vi "Update Settings button colors.vi"(7 "Host":T1, 8 "error in (no error)":errorcluster, 9 "Force Default Colors (F)":bool, 10 "Bool Refnum":refnum<vi>, 11 "Settings in":T4) -> (0 "error out":errorcluster, 3 "Settings out":T4)   [LabVIEW 2021]
doc: "Change the colors of the boolean button according to Settings in and Host in. Consider whether the data log file will be overwritten: default colors when safe, red tint when overwriting. Otherwise, consider whether there are no IO resources: default colors when present, yellow tint when missing."
uses:
  Settings/Settings.lvlib
  Acquisition/IO Device.ctl
  Acquisition/Acquisition.lvlib
  Acquisition/Channel Settings.ctl
  Interval Timer/Interval Length.ctl
  Interval Timer/Interval Timer.lvlib
  Interval Timer/Repeat Interval.ctl
  Interval Timer/Interval Token.ctl
  Acquisition/Hardware Configuration.ctl
  Logging/Logging Configuration.ctl
  Logging/Logging.lvlib
  Diagnostics/Diagnostics Configuration.ctl
  Diagnostics/Diagnostics.lvlib
  Settings/Settings.ctl
  Acquisition/Host Software Package.ctl
  Acquisition/Host IO Resource.ctl
  Acquisition/Host Resources.ctl
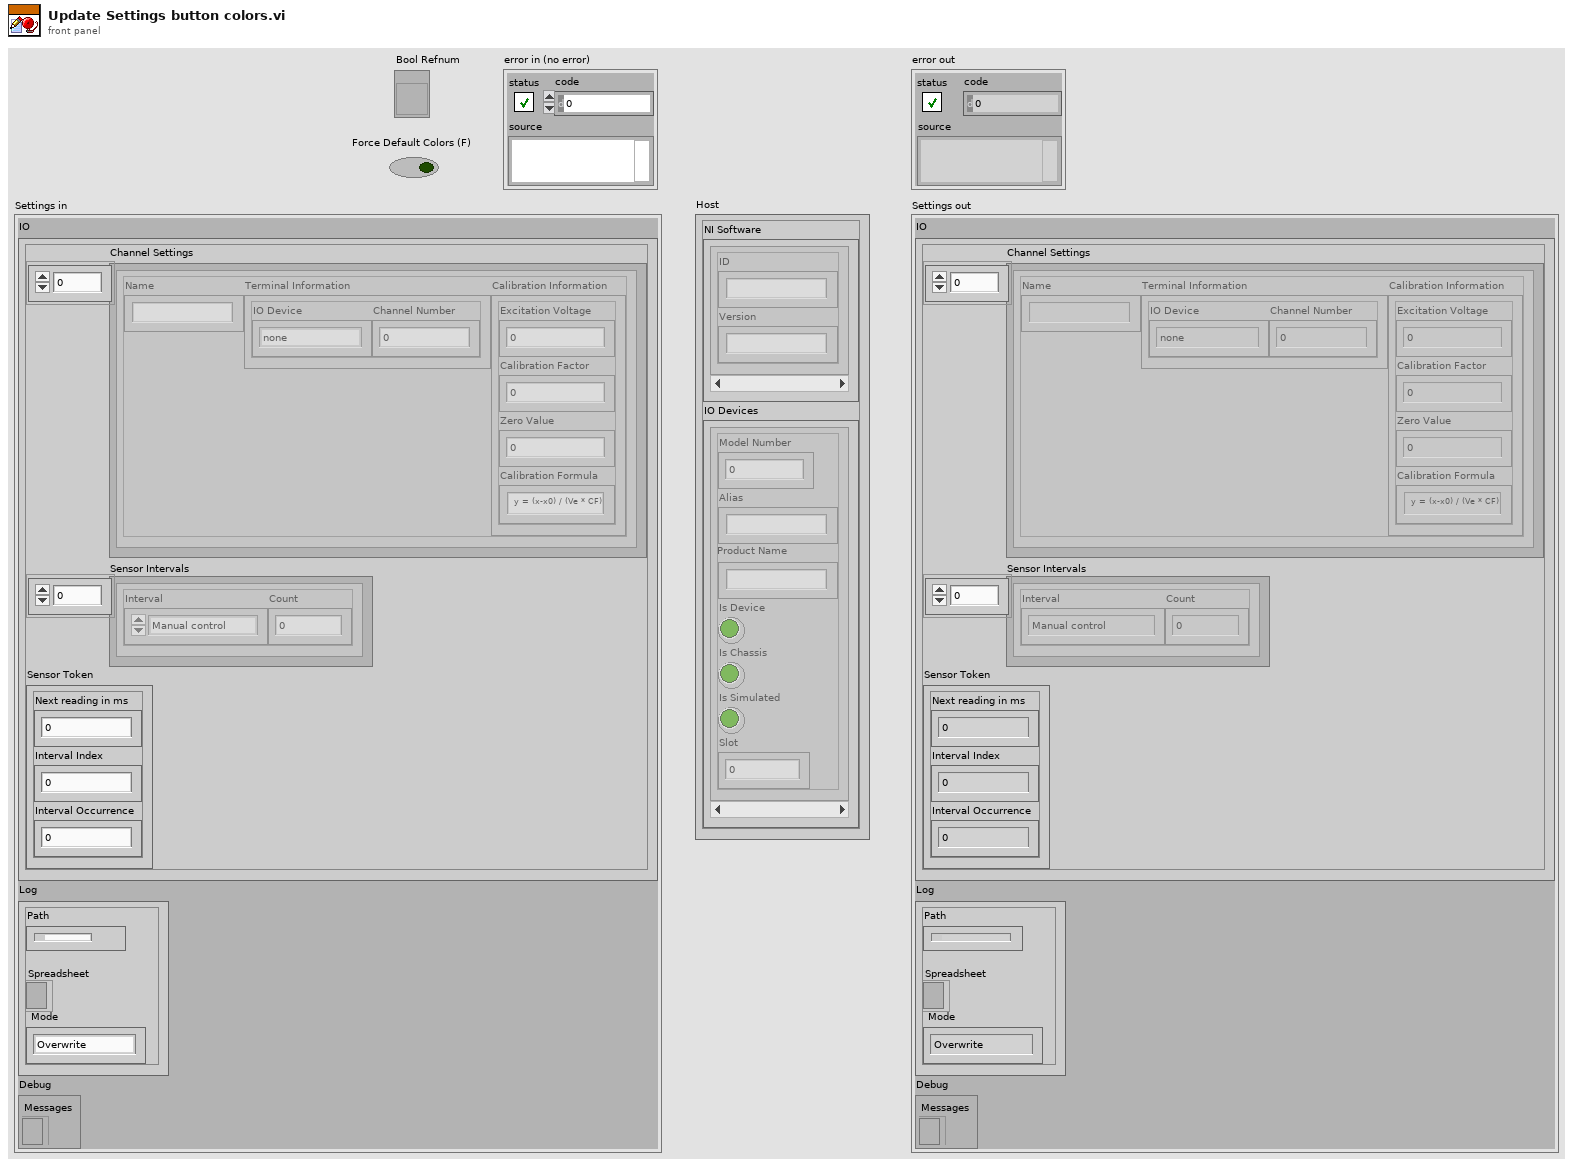
[diagram p1: front panel]
types:
  T1 = typedef "Acquisition.lvlib/Host Resources.ctl" = cluster{"NI Software":T2[], "IO Devices":T3[]}
  T2 = typedef "Acquisition.lvlib/Host Software Package.ctl" = cluster{"ID":string, "Version":string}
  T3 = typedef "Acquisition.lvlib/Host IO Resource.ctl" = cluster{"Model Number":u32, "Alias":string, "Product Name":string, "Is Device":bool, "Is Chassis":bool, "Is Simulated":bool, "Slot":i32}
  T4 = typedef "Settings.lvlib/Settings.ctl" = cluster{"IO":T5, "Log":T11, "Debug":T12}
  T5 = typedef "Acquisition.lvlib/Hardware Configuration.ctl" = cluster{"Channel Settings":T6[], "Sensor Intervals":T8[], "Sensor Token":T10}
  T6 = typedef "Acquisition.lvlib/Channel Settings.ctl" = cluster{"Name":string, "Terminal Information":cluster{"IO Device":T7, "Channel Number":i32}, "Calibration Information":cluster{"Excitation Voltage":dbl, "Calibration Factor":dbl, "Zero Value":dbl, "Calibration Formula":string}}
  T7 = typedef "Acquisition.lvlib/IO Device.ctl" = enum16{"none", "9219", "9401"}
  T8 = typedef "Interval Timer.lvlib/Repeat Interval.ctl" = cluster{"Interval":T9, "Count":i32}
  T9 = typedef "Interval Timer.lvlib/Interval Length.ctl" = enum16{"Manual control", "1 second", "10 seconds", "30 seconds", "60 seconds", "600 seconds", "1200 seconds", "3600 seconds"}
  T10 = typedef "Interval Timer.lvlib/Interval Token.ctl" = cluster{"Next reading in ms":u32, "Interval Index":i32, "Interval Occurrence":i32}
  T11 = typedef "Logging.lvlib/Logging Configuration.ctl" = cluster{"Path":path, "Spreadsheet":refnum<file>, "Mode":enum16{"Overwrite", "Append", "Create New"}}
  T12 = typedef "Diagnostics.lvlib/Diagnostics Configuration.ctl" = cluster{"Messages":refnum<file>}
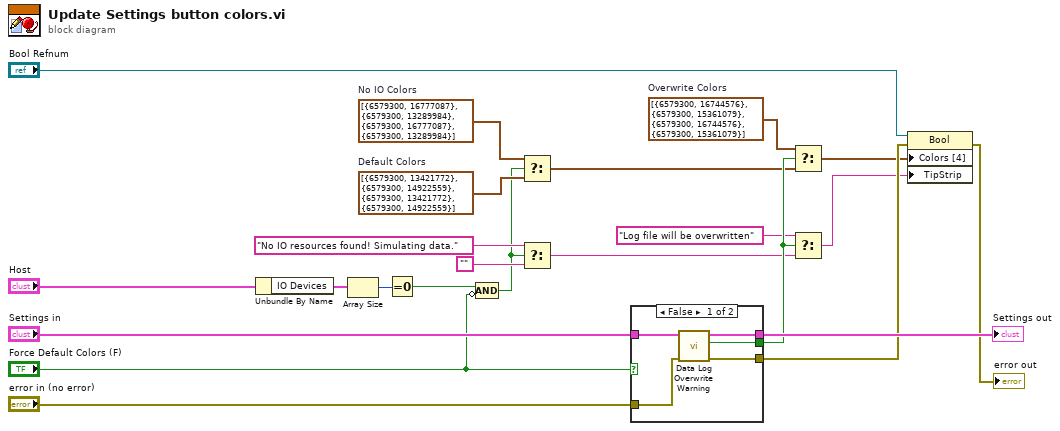
[diagram p0: block diagram]
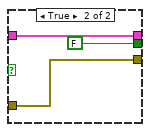
[diagram p2: hidden frame]
diagram:
  w7 = cluster{"Color Box":u32, "Color Box 2":u32}[] [{"Color Box"=6579300, "Color Box 2"=16777087}, {"Color Box"=6579300, "Color Box 2"=13289984}, {"Color Box"=6579300, "Color Box 2"=16777087}, {"Color Box"=6579300, "Color Box 2"=13289984}]  # No IO Colors
  w8 = cluster{"Color Box":u32, "Color Box 2":u32}[] [{"Color Box"=6579300, "Color Box 2"=13421772}, {"Color Box"=6579300, "Color Box 2"=14922559}, {"Color Box"=6579300, "Color Box 2"=13421772}, {"Color Box"=6579300, "Color Box 2"=14922559}]  # Default Colors
  w20 = cluster{"Color Box":u32, "Color Box 2":u32}[] [{"Color Box"=6579300, "Color Box 2"=16744576}, {"Color Box"=6579300, "Color Box 2"=15361079}, {"Color Box"=6579300, "Color Box 2"=16744576}, {"Color Box"=6579300, "Color Box 2"=15361079}]  # Overwrite Colors
  n1 = Unbundle By Name("Host") -> ("IO Devices"=w11:T3[])
  n2 = Array Size(array=w11) -> (size(s)=w4:i32)
  n3 = Equal To 0?(x=w4) -> (x = 0?=w2:bool)
  n4 = Compound Arithmetic op=AND(w2, invert "Force Default Colors (F)") -> (w1:bool)
  n5 = Select(t=w7, s=w1, f=w8) -> (s? t:f=w6:cluster{"Color Box":u32, "Color Box 2":u32}[])
  n6 = Select(t="No IO resources found! Simulating data.", s=w1, f="") -> (s? t:f=w5:string)
  n7 = case shown="False" "Force Default Colors (F)" {
    tunnel: "Settings in" -> [w28 w29]
    tunnel: [w27 w29] -> w22
    tunnel: "error in (no error)" -> [w26 w30]
    tunnel: [w25 w30] -> w18
    tunnel: [w24 FALSE ("Overwrite Warning?")] -> w15
    frame False {
      n8 = call "Data Log Overwrite Warning.vi"("error in (no error)"=w26, "Settings in"=w28) -> ("error out"=w25:errorcluster, "Overwrite Warning?"=w24:bool, "Settings out"=w27:T4)  [unwired: 7 in]
    }
    frame True {
    }
  }
  "Settings out" <- w22
  n9 = Select(t=w20, s=w15, f=w6) -> (s? t:f=w16:cluster{"Color Box":u32, "Color Box 2":u32}[])
  n10 = Select(t="Log file will be overwritten", s=w15, f=w5) -> (s? t:f=w13:string)
  n11 = property class="Bool"(reference="Bool Refnum", error in=w18, "Colors [4]"=w16, "TipStrip"=w13) -> (error out=→"error out":errorcluster)  [unwired: 1 out]
